vi "sv_Overall Level (N Channels).vi"(0 "even-angle signals":cluster{"r0":dbl, "dr":dbl, "Y":dbl[]}[](array[cluster]) {"r0" format="%.2p"; "dr" format="%.2p"; "Y" format="%.2f"}, 1 "x-axis selection":u16(ring)=2 items=["Time", "Revolution", "Frequency"], 2 "reset? (F)":bool, 5 "even-angle channel info":T3[](array[typedef]) {"channel info"."pregain" format="%.2f"; "channel info"."weighting filter" items=["Linear", "A-weighting", "B-weighting", "C-weighting", "ITU-R 468-4", "Dolby", "CCITT", "C-message", "Wb", "Wc", "Wd", "We", "Wf", "Wh", "Wj", "Wk", "Wm", "AES17 20 kHz lowpass", "AES17 40 kHz lowpass", "AES17 20 kHz highpass", "AES17 40 kHz highpass"]; "channel info"."dB reference" format="%^.1e"; "channel info"."engineering units" items=["custom..."=0, "V"=1, "A"=21, "C"=30, "pC"=31, "s"=32, "-"=29, "Pa"=2, "N"=20, "g"=3, "m/s^2"=4, "m/s"=5, "m"=6, "mm/s"=12, "mm"=13, "micron/s"=14, "micron"=15, "in/s^2"=7, "in/s"=8, "in"=9, "mil/s"=10, "mil"=11, "rad/s^2"=16, "rad/s"=17, "rad"=18, "deg/s^2"=26, "deg/s"=27, "deg"=28, "RPM"=22, "cycle/s^2"=23, "Hz"=24, "cycle"=25, "strain"=19]; "channel info"."sensor sensitivity" format="%#_5f"}, 7 "even-angle position info":T1, 9 "dB on? (F)":bool, 11 "error in (no error)":errorcluster, 12 "integration revolution":dbl=1.0) -> (4 "overall levels":cluster{"time/rev/rpm":dbl[], "level":dbl[]}[](array[cluster]), 6 "unit labels":T2(array[cluster]), 8 "level position info":T1, 15 "error out":errorcluster)   [LabVIEW 2017, in "SoundVib_ContSweptSine.lvlib"]
doc: "Computes the root-mean-square (RMS) level of the <B>even-angle signal</B> and generates an XY graph as the output. The data type you wire to the <B>even-angle signal</B> input determines the polymorphic instance to use."
uses:
  <vilib>/addons/Sound and Vibration/svt_Continuous Swept Sine/SoundVib_ContSweptSine.lvlib
  <vilib>/addons/Sound and Vibration/Order Analysis/Misc/OAT Position Info.ctl
  <vilib>/addons/_NISVFA/_Shared subVIs/Controls/svc_Resampled Channel Info.ctl
  <vilib>/addons/_NISVFA/_Shared subVIs/Controls/svc_Channel Info.ctl
  <vilib>/addons/_NISVFA/_Shared subVIs/Controls/svc_Engineering Units Text Ring.ctl
  <vilib>/addons/_NISVFA/_Shared subVIs/Controls/svc_Weighting Filter Text Ring.ctl
  <vilib>/addons/Sound and Vibration/Order Analysis/Resample Order Tracking/SoundVib_Resampling.lvlib
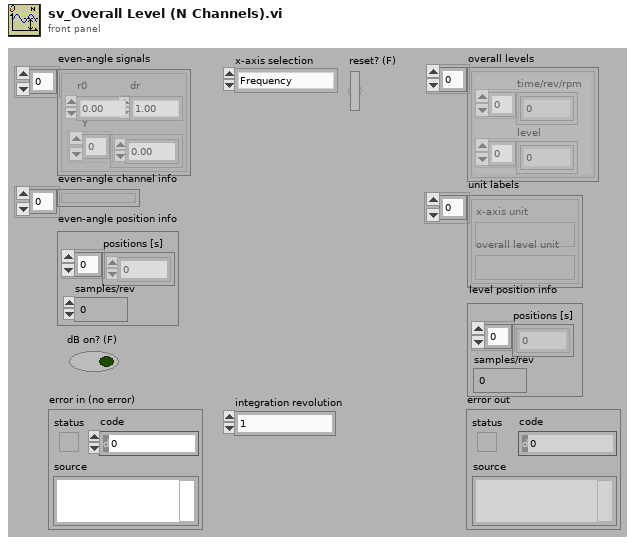
[diagram p1: front panel]
types:
  T1 = typedef "OAT Position Info.ctl" = cluster{"positions [s]":dbl[], "samples/rev":dbl}
  T2 = cluster{"x-axis unit":string, "overall level unit":string}[]
  T3 = typedef "svc_Resampled Channel Info.ctl" = cluster{"channel name":string, "description":string, " channel info":T4}
  T4 = typedef "svc_Channel Info.ctl" = cluster{"sensor sensitivity":dbl, "engineering units":T5, "dB reference":dbl, "custom label":string, "weighting filter":T6, "pregain":dbl}
  T5 = typedef "svc_Engineering Units Text Ring.ctl" = u16
  T6 = typedef "svc_Weighting Filter Text Ring.ctl" = u16
  T7 = typedef "SoundVib_TachProcess.lvlib/speed profile.ctl" = cluster{"time [s]":dbl[], "speed [RPM]":dbl[]}
  T8 = cluster{"X axis unit":string, "overall level unit":string}[]
  T9 = cluster{"time/rev/rpm":dbl[], "magnitude":dbl[]}[]
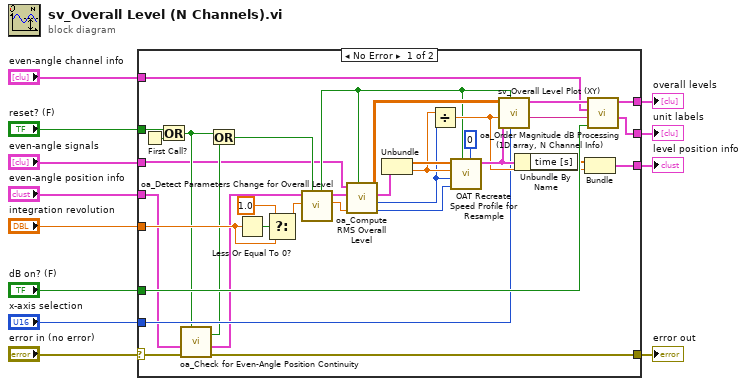
[diagram p0: block diagram]
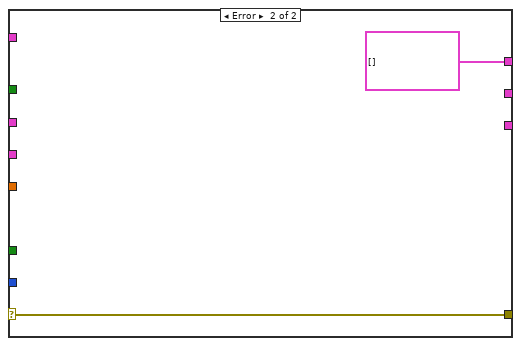
[diagram p2: hidden frame]
diagram:
  n1 = case shown="No Error" "error in (no error)" {
    selector: "error in (no error)" -> [w18 w49]
    tunnel: [w17 w49] -> w11
    tunnel: "even-angle signals" -> [w16 _]
    tunnel: "even-angle position info" -> [w14 _]
    tunnel: "integration revolution" -> [w28 _]
    tunnel: "reset? (F)" -> [w25 _]
    tunnel: [w41 cluster{"X":dbl[], "Y":dbl[]}[] [] ("magnitudes")] -> w6
    tunnel: "dB on? (F)" -> [w40 _]
    tunnel: "even-angle channel info" -> [w15 _]
    tunnel: [w36 _] -> w3
    tunnel: "x-axis selection" -> [w33 _]
    tunnel: [w31 _] -> w1
    frame No Error {
      n2 = First Call?() -> (First Call?: T/F=w26:bool)
      n3 = Or(x=w25, y=w26) -> (x .or. y?=w21:bool)
      n4 = call <vilib>:"oa_Check for Even-Angle Position Continuity.vi"("reset in"=w21, "error in (no error)"=w18, "even-angle position info"=w14) -> ("error out"=w17:errorcluster, "even-angle position info dup"=w13:T1, "position not continuous"=w20:bool)  [unwired: 6 in]
      n5 = Or(x=w21, y=w20) -> (x .or. y?=w19:bool)
      n6 = Less Or Equal To 0?(x=w28) -> (x <= 0?=w30:bool)
      n7 = Select(t=1.0, s=w30, f=w28) -> (s? t:f=w27:dbl)
      n8 = call <vilib>:"oa_Detect Parameters Change for Overall Level.vi"("reset (F)"=w19, "integration revolution"=w27, "even angle position info"=w13) -> ("dup integration revolution"=w22:dbl, "dup even angle position"=w23:T1, "reset out"=w24:bool)  [unwired: 6 in]
      n9 = call <vilib>:"oa_Compute RMS Overall Level.vi"("reset"=w24, "integration revolution"=w22, "even angle position info in"=w23, "even angle signals"=w16) -> ("output length"=w45:i32, "decimation factor"=w34:i32, "even angle position info out"=w35:T1, "output RMS level"=w44:dbl[][])  [unwired: 4 in]
      n10 = Unbundle(w35) -> ("positions [s]"=w47:dbl[], "samples/rev"=w46:dbl)
      n11 = Divide(x=w46, y=w34) -> (x/y=w37:dbl)
      n12 = call <vilib>:"OAT Recreate Speed Profile for Resample.vi"("lags"=0, "init/continue (init:T)"=w24, "output length"=w45, "decimation factor"=w34, "sample / rev"=w46, "time stamps in"=w47) -> ("speed profile"=w39:T7)  [unwired: 5 in]
      n13 = call <vilib>:"sv_Overall Level Plot (XY).vi"("X axis selection"=w33, "reset? (True)"=w24, "speed profile"=w39, "samples/rev"=w37, "overall level (even angular)"=w44) -> ("X unit"=w32:string, "overall level"=w42:cluster{"X":dbl[], "Y":dbl[]}[])  [unwired: 5 in]
      n14 = Unbundle By Name(w39) -> ("time [s]"=w38:dbl[])
      n15 = Bundle("time [s]"=w38, w37) -> (w36:cluster{"time [s]":dbl[], dbl})  [unwired: 1 in]
      n16 = call <vilib>:"oa_Order Magnitude dB Processing (1D array, N Channel Info).vi"("dB on? (T)"=w40, "x axis unit label"=w32, "even angle channel info"=w15, "magnitudes"=w42) -> ("unit labels"=w31:T8, "magnitudes dB"=w41:T9)  [unwired: 6 in]
    }
    frame Error {
    }
  }
  "error out" <- w11
  "overall levels" <- w6
  "unit labels" <- w1
  "level position info" <- w3
